vi "mxwScript_API_XMLTemplateName_AddDropRelation.vi"(7 "direction":T1, 8 "error in (no error)":errorcluster, 9 "addWireSpace":bool=TRUE, 10 "distance":i32 min=0, 11 "absolutePath":string) -> (0 "error out":errorcluster, 3 "encoded absolutePath":string)   [LabVIEW 2020]
doc: "Add diagram to drop this template into to the template name."
uses:
  codeGenAPISupport.llb/cgAPI_mxwScript_DrpTmplt_SimpleDirection.ctl
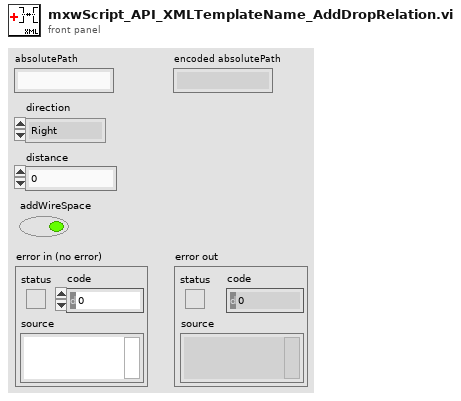
[diagram p1: front panel]
types:
  T1 = typedef "cgAPI_mxwScript_DrpTmplt_SimpleDirection.ctl" = enum16{"Right", "Left", "Below", "Above"}
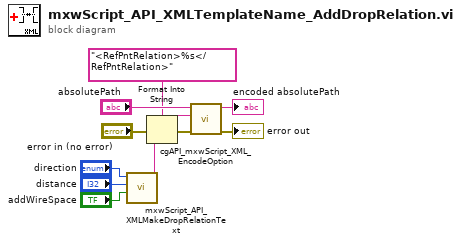
[diagram p0: block diagram]
diagram:
  n1 = call "mxwScript_API_XMLMakeDropRelationText.vi"("addWireSpace"="addWireSpace", "distance"="distance", "direction"="direction") -> ("XML out"=w4:string)  [unwired: 8 out]
  n2 = Format Into String(format string="<RefPntRelation>%s</RefPntRelation>" ("control name"), error in="error in (no error)", w4) -> (resulting string=w6:string, error out=w8:errorcluster)  [unwired: 1 in]
  n3 = call "cgAPI_mxwScript_XML_EncodeOption.vi"("error in (no error)"=w8, "otherXML"=w6, "normalTextString"="absolutePath") -> ("error out"=→"error out":errorcluster, "encodedString"=→"encoded absolutePath":string)  [unwired: 7 out]
